vi "Database.SearchForNewFiles.vi"(8 "error in":errorcluster) -> (0 "error out":errorcluster)   [LabVIEW 2016]
uses:
  Global/ApplicationGlobal.vi
  Logger/Logger.FileBody.ctl
panel:
  out "HandledFileContent":T1[](array[typedef]) {"Values" format="%.3f"}
  out "HandledFileContent":T1 {"Values" format="%.3f"}
  out "Array":string[](array[string])
  out "text":string
  in  "ResultsFile":u32[](array[numeric])
  out "SerialNo":string
  out "Variant":string
  out "System":string
  out "filenames":string[](array[string])
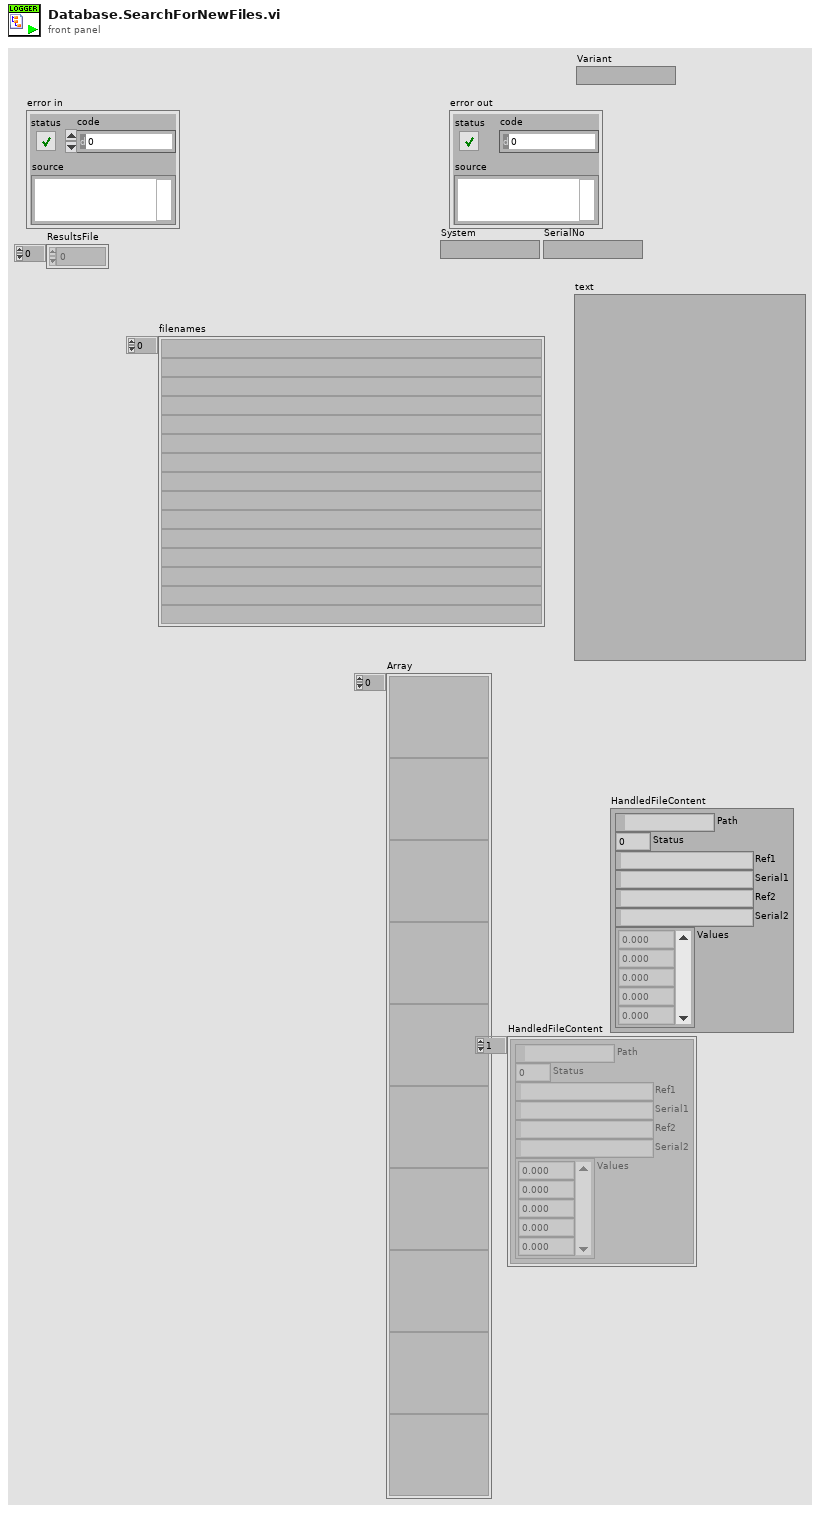
[diagram p1: front panel]
types:
  T1 = typedef "Logger.FileBody.ctl" = cluster{"Path":path, "Status":u8, "Ref1":string, "Serial1":string, "Ref2":string, "Serial2":string, "Values":sgl[]}
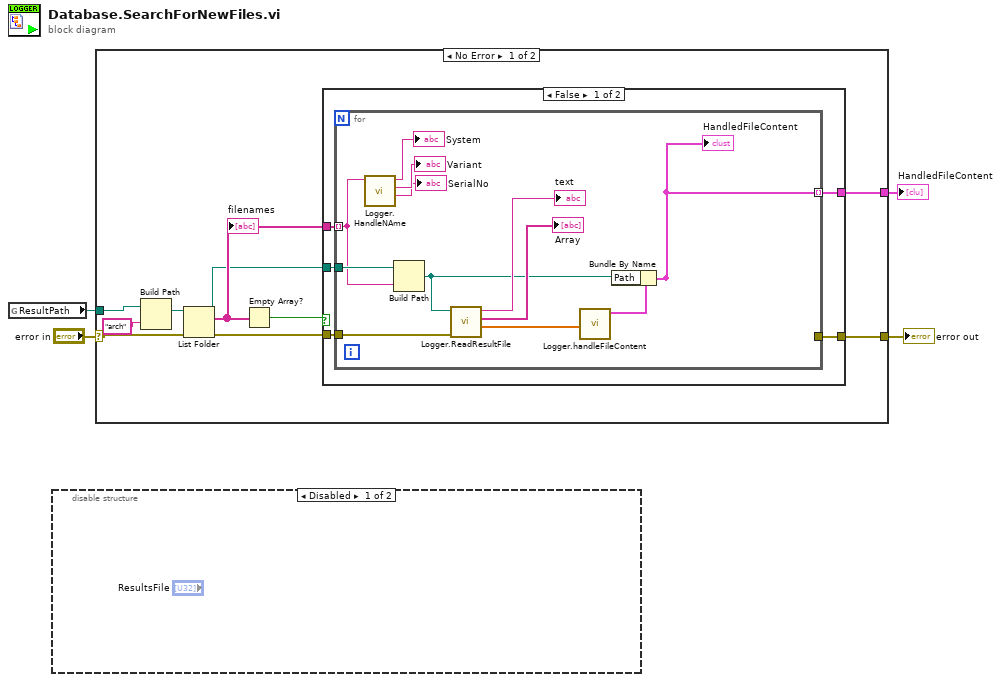
[diagram p0: block diagram]
diagram:
  n1 = global read "ApplicationGlobal.vi" "ResultPath"() -> (w2:path)
  n2 = disable-structure shown="Disabled" {
    frame Disabled {
    }
    frame Enabled {
    }
  }
  n3 = case shown="No Error" "error in" {
    selector: "error in" -> [w14 w35]
    tunnel: [w8 w35] -> w4
    tunnel: w2 -> [w7 _]
    tunnel: [w10 _] -> w1
    frame No Error {
      n4 = Build Path(base path=w7, name or relative path="arch") -> (appended path=w5:path)
      n5 = List Folder(path=w5, error in=w14) -> (path out=w11:path, filenames=w12:string[], error out=w9:errorcluster)  [unwired: 2 in, 1 out]
      "filenames" <- w12
      n6 = Empty Array?(array=w12) -> (empty?=w13:bool)
      n7 = case shown="False" w13 {
        tunnel: w12 -> [w19 _]
        tunnel: w11 -> [w18 _]
        tunnel: [w17 _] -> w10
        tunnel: w9 -> [w16 w34]
        tunnel: [w15 w34] -> w8
        frame False {
          n8 = for {
            tunnel: w19 -> [w29] mode=indexing
            tunnel: w18 -> [w30]
            tunnel: [w21] -> w17 mode=indexing
            tunnel: w16 -> [w25]
            tunnel: [w23] -> w15
            n9 = call "Logger.HandleNAme.vi"("String"=w29) -> ("SerialNo"=→"SerialNo":string, "Variant"=→"Variant":string, "System"=→"System":string)  [unwired: 8 in]
            n10 = Build Path(base path=w30, name or relative path=w29) -> (appended path=w20:path)
            n11 = call "Logger.ReadResultFile.vi"("error in"=w25, "ResultFilePath"=w20) -> ("error out"=w24:errorcluster, 1:"ResultValues"=w28:dbl[], 2:"ResultValues"=→"Array":string[], "text"=→"text":string)  [unwired: 6 in]
            n12 = call "Logger.handleFileContent.vi"("ResultsFile"=w28) -> ("HandledFileContent"=w22:T1)  [unwired: 10 in]
            n13 = Bundle By Name(cluster=w22, "Path"=w20) -> (w21:T1)
            "HandledFileContent" <- w21
          }
        }
        frame True {
        }
      }
    }
    frame Error {
    }
  }
  "error out" <- w4
  "HandledFileContent" <- w1
